vi "Untitled 3.vi"() -> ()   [LabVIEW 2019]
uses:
  <vilib>/rvi/Emulation/niFpgaGetClockAttributes.vi
  <vilib>/rvi/Emulation/niFpgaSctlEmulationGetInTimedLoop.vi
  <vilib>/rvi/Emulation/niFpgaEmulationReportErrorSimple.vi
  <vilib>/rvi/eio/common/nirviEmuTemplateMethod_errors.vi
  <vilib>/rvi/Emulation/niFpgaCriticalErrorInLSC.vi
  <vilib>/eio/EIONode/EIONode.xnode
panel:
  out "Tick Count(mSec) 2":u32 caption="Tick Count(mSec)"
  in  "Count(mSec)":u32
  in  "Sample":bool
  out "Period":u32
  out "Count":i16
  out "Time":u32 format="%<%H:%M>t"
  out "DI2 2":i16
  out "DI0 2":i16
  out "DI1 2":i16
  out "Mod8/DI1 2":bool
  out "Mod8/DI2 2":bool
  out "Mod8/DI0 2":bool
  out "Count 1":i16
  out "Mod8/DI0":bool
  out "Mod8/DI2":bool
  out "Mod8/DI1":bool
  out "DI1":i16
  out "DI0":i16
  out "DI2":i16
  in  "stop":bool
  out "Position":i16
  in  "Reset":bool
  out "RPM":u32
  out "Count1":u32
  out "Tick Count(mSec)":u32
  out "Umdrehung":i32
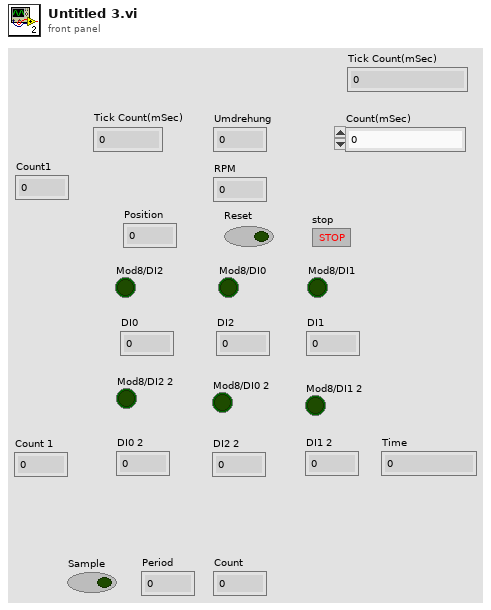
[diagram p1: front panel]
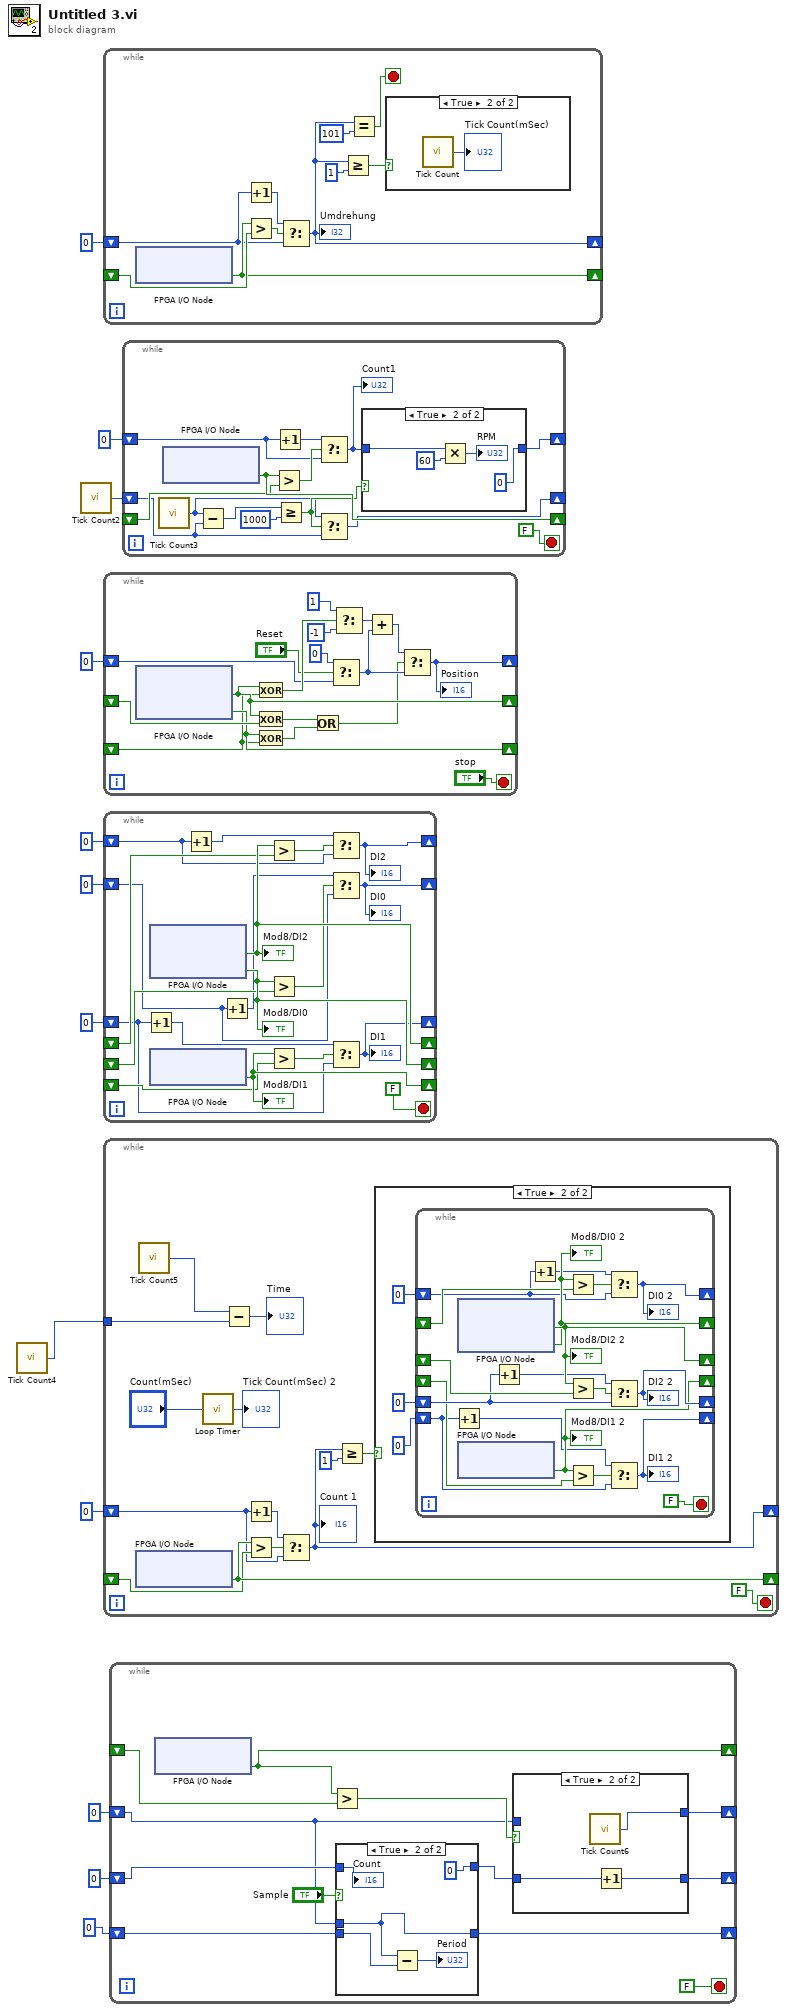
[diagram p0: block diagram]
diagram:
  n1 = call "Tick Count4"() -> ("Tick Count(mSec)"=w4:u32)
  n2 = call "Tick Count2"() -> ("Tick Count(mSec)"=w11:u32)
  n3 = while {
    shift-right: [w21] -> _
    shift-left: _ -> [w22]
    shift-right: [w15] -> _
    shift-left: 0 ("x") -> [w18]
    stop <- w16 stop-if-true
    n4 = xnode "FPGA I/O Node"() -> ("Mod8/DI1"=w21:bool)  [unwired: 1 in, 1 out]
    n5 = Increment(x=w18) -> (x+1=w20:i32)
    n6 = Greater?(x=w21, y=w22) -> (0:w19:bool)
    n7 = Select(t=w20, s=w19, f=w18) -> (s? t:f=w15:i32)
    "Umdrehung" <- w15
    n8 = Greater Or Equal?(x=w15, y=1) -> (x >= y?=w13:bool)
    n9 = Equal?(x=w15, y=101) -> (x = y?=w16:bool)
    n10 = case shown="True" w13 {
      frame False {
      }
      frame True {
        n11 = call "Tick Count"() -> ("Tick Count(mSec)"=→"Tick Count(mSec)":u32)
      }
    }
  }
  n12 = while {
    shift-right: [w39] -> _
    shift-left: _ -> [w41]
    shift-right: [w40] -> _
    shift-left: _ -> [w38]
    shift-right: [w26] -> _
    shift-left: i16 0 ("t") -> [w30]
    stop <- "stop" stop-if-true
    n13 = xnode "FPGA I/O Node"() -> ("Mod8/DI2"=w39:bool, "Mod8/DI0"=w40:bool)  [unwired: 2 in, 2 out]
    n14 = Exclusive Or(1:w38, 2:w39) -> (0:w35:bool)
    n15 = Exclusive Or(1:w41, 2:w39) -> (0:w37:bool)
    n16 = Exclusive Or(1:w38, 2:w40) -> (0:w36:bool)
    n17 = Or(x=w37, y=w36) -> (x .or. y?=w25:bool)
    n18 = Select(t=i16 0, s="Reset", f=w30) -> (s? t:f=w28:i16)
    n19 = Select(t=i16 1, s=w35, f=i16 -1) -> (s? t:f=w32:i16)
    n20 = Add(x=w32, y=w28) -> (x+y=w29:i16)
    n21 = Select(t=w29, s=w25, f=w28) -> (s? t:f=w26:i16)
    "Position" <- w26
  }
  n22 = while {
    shift-right: [w60] -> _
    shift-left: _ -> [w59]
    shift-right: [w58] -> _
    shift-left: _ -> [w57]
    shift-right: [w54] -> _
    shift-left: i16 0 ("x") -> [w55]
    shift-right: [w51] -> _
    shift-left: i16 0 ("x") -> [w50]
    shift-right: [w48] -> _
    shift-left: _ -> [w47]
    shift-right: [w45] -> _
    shift-left: i16 0 ("x") -> [w44]
    stop <- FALSE stop-if-true
    n23 = Increment(x=w44) -> (x+1=w46:i16)
    n24 = xnode "FPGA I/O Node"() -> ("Mod8/DI2"=w60:bool, "Mod8/DI0"=w58:bool)  [unwired: 2 in, 2 out]
    "Mod8/DI2" <- w60
    "Mod8/DI0" <- w58
    n25 = xnode "FPGA I/O Node"() -> ("Mod8/DI1"=w48:bool)  [unwired: 1 in, 1 out]
    "Mod8/DI1" <- w48
    n26 = Increment(x=w55) -> (x+1=w56:i16)
    n27 = Increment(x=w50) -> (x+1=w52:i16)
    n28 = Greater?(x=w60, y=w59) -> (0:w53:bool)
    n29 = Greater?(x=w58, y=w57) -> (0:w49:bool)
    n30 = Greater?(x=w48, y=w47) -> (0:w42:bool)
    n31 = Select(t=w56, s=w53, f=w55) -> (s? t:f=w54:i16)
    "DI2" <- w54
    n32 = Select(t=w52, s=w49, f=w50) -> (s? t:f=w51:i16)
    "DI0" <- w51
    n33 = Select(t=w46, s=w42, f=w44) -> (s? t:f=w45:i16)
    "DI1" <- w45
  }
  n34 = while {
    shift-right: [w74] -> _
    shift-left: _ -> [w73]
    shift-right: [w68] -> _
    shift-left: i16 0 ("x") -> [w70]
    tunnel: w4 -> [w64]
    stop <- FALSE stop-if-true
    n35 = xnode "FPGA I/O Node"() -> ("Mod8/DI1"=w74:bool)  [unwired: 1 in, 1 out]
    n36 = call "Tick Count5"() -> ("Tick Count(mSec)"=w65:u32)
    n37 = call "Loop Timer"("Count(mSec)"="Count(mSec)") -> ("Tick Count(mSec)"=→"Tick Count(mSec) 2":u32)
    n38 = Subtract(x=w65, y=w64) -> (x-y=→"Time":u32)
    n39 = Increment(x=w70) -> (x+1=w71:i16)
    n40 = Greater?(x=w74, y=w73) -> (0:w72:bool)
    n41 = Select(t=w71, s=w72, f=w70) -> (s? t:f=w68:i16)
    "Count 1" <- w68
    n42 = Greater Or Equal?(x=w68, y=i16 1 ("x")) -> (x >= y?=w67:bool)
    n43 = case shown="True" w67 {
      frame False {
      }
      frame True {
        n44 = while {
          shift-right: [w96] -> _
          shift-left: _ -> [w95]
          shift-right: [w94] -> _
          shift-left: _ -> [w93]
          shift-right: [w90] -> _
          shift-left: i16 0 -> [w91]
          shift-right: [w87] -> _
          shift-left: i16 0 -> [w86]
          shift-right: [w84] -> _
          shift-left: _ -> [w83]
          shift-right: [w81] -> _
          shift-left: i16 0 -> [w80]
          stop <- FALSE stop-if-true
          n45 = Increment(x=w80) -> (x+1=w82:i16)
          n46 = xnode "FPGA I/O Node"() -> ("Mod8/DI2"=w96:bool, "Mod8/DI0"=w94:bool)  [unwired: 2 in, 2 out]
          "Mod8/DI2 2" <- w96
          "Mod8/DI0 2" <- w94
          n47 = xnode "FPGA I/O Node"() -> ("Mod8/DI1"=w84:bool)  [unwired: 1 in, 1 out]
          "Mod8/DI1 2" <- w84
          n48 = Increment(x=w91) -> (x+1=w92:i16)
          n49 = Increment(x=w86) -> (x+1=w88:i16)
          n50 = Greater?(x=w94, y=w93) -> (0:w85:bool)
          n51 = Greater?(x=w96, y=w95) -> (0:w89:bool)
          n52 = Greater?(x=w84, y=w83) -> (0:w78:bool)
          n53 = Select(t=w88, s=w85, f=w86) -> (s? t:f=w87:i16)
          "DI0 2" <- w87
          n54 = Select(t=w92, s=w89, f=w91) -> (s? t:f=w90:i16)
          "DI2 2" <- w90
          n55 = Select(t=w82, s=w78, f=w80) -> (s? t:f=w81:i16)
          "DI1 2" <- w81
        }
      }
    }
  }
  n56 = while {
    shift-right: [w108] -> _
    shift-left: _ -> [w107]
    shift-right: [w105] -> _
    shift-left: u32 0 ("Tick Count(mSec)") -> [w101]
    shift-right: [w103] -> _
    shift-left: i16 0 ("x") -> [w102]
    shift-right: [w99] -> _
    shift-left: u32 0 ("y") -> [w100]
    stop <- FALSE stop-if-true
    n57 = xnode "FPGA I/O Node"() -> ("Mod8/DI1"=w108:bool)  [unwired: 1 in, 1 out]
    n58 = Greater?(x=w108, y=w107) -> (0:w106:bool)
    n59 = case shown="True" "Sample" {
      tunnel: [w110 i16 0 ("x")] -> w104
      tunnel: w102 -> [w110 w114]
      tunnel: w101 -> [_ w112]
      tunnel: w100 -> [w109 w113]
      tunnel: [w109 w112] -> w99
      frame False {
      }
      frame True {
        n60 = Subtract(x=w112, y=w113) -> (x-y=→"Period":u32)
        "Count" <- w114
      }
    }
    n61 = case shown="True" w106 {
      tunnel: [w117 w120] -> w105
      tunnel: w101 -> [w117 _]
      tunnel: w104 -> [w116 w119]
      tunnel: [w116 w118] -> w103
      frame False {
      }
      frame True {
        n62 = call "Tick Count6"() -> ("Tick Count(mSec)"=w120:u32)
        n63 = Increment(x=w119) -> (x+1=w118:i16)
      }
    }
  }
  n64 = while {
    shift-right: [w134] -> _
    shift-left: _ -> [w133]
    shift-right: [w123] -> _
    shift-left: w11 -> [w122]
    shift-right: [w124] -> _
    shift-left: u32 0 ("x") -> [w125]
    stop <- FALSE stop-if-true
    n65 = call "Tick Count3"() -> ("Tick Count(mSec)"=w121:u32)
    n66 = xnode "FPGA I/O Node"() -> ("Mod8/DI1"=w134:bool)  [unwired: 1 in, 1 out]
    n67 = Subtract(x=w121, y=w122) -> (x-y=w130:u32)
    n68 = Greater?(x=w134, y=w133) -> (0:w132:bool)
    n69 = Increment(x=w125) -> (x+1=w131:u32)
    n70 = Greater Or Equal?(x=w130, y=u32 1000) -> (x >= y?=w126:bool)
    n71 = Select(t=w131, s=w132, f=w125) -> (s? t:f=w128:u32)
    "Count1" <- w128
    n72 = Select(t=w121, s=w126, f=w122) -> (s? t:f=w123:u32)
    n73 = case shown="True" w126 {
      tunnel: w128 -> [w135 w136]
      tunnel: [w135 u32 0 ("Tick Count(mSec)")] -> w124
      frame False {
      }
      frame True {
        n74 = Multiply(x=w136, y=u32 60) -> (x*y=→"RPM":u32)
      }
    }
  }
